vi "DB_Write.vi"(0 "Input Params":T1={"Address IP"="192.168.1.12", "Rack"=0, "Slot "=2, "DB Number"=1, "Start"=0, "Amount"=0, "Word Length"=2} {"Word Length" items=["Bit"=1, "Byte"=2, "Word"=4, "DWord"=6, "Real"=8, "Counter"=28, "Timer"=29]}, 7 "Array":u8[](array[numeric])) -> (15 "Status":string="No Error")   [LabVIEW 2023]
uses:
  snap7-full-1.4.0/LabVIEW/lib/Snap7.lvlib
panel:
  out "?":string
  out "Running":bool
  in  "?":bool
  # "DB Fill"
  # "WARNING !!!\nThis program will fill a DB Entirely"
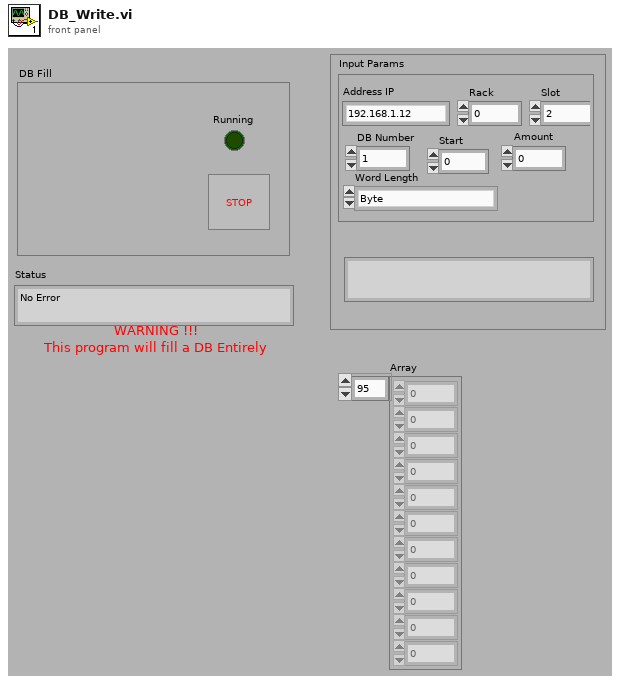
[diagram p1: front panel]
types:
  T1 = cluster{"Address IP":string, "Rack":i32, "Slot ":i32, "DB Number":i32, "Start":i32, "Amount":i32, "Word Length":i32}
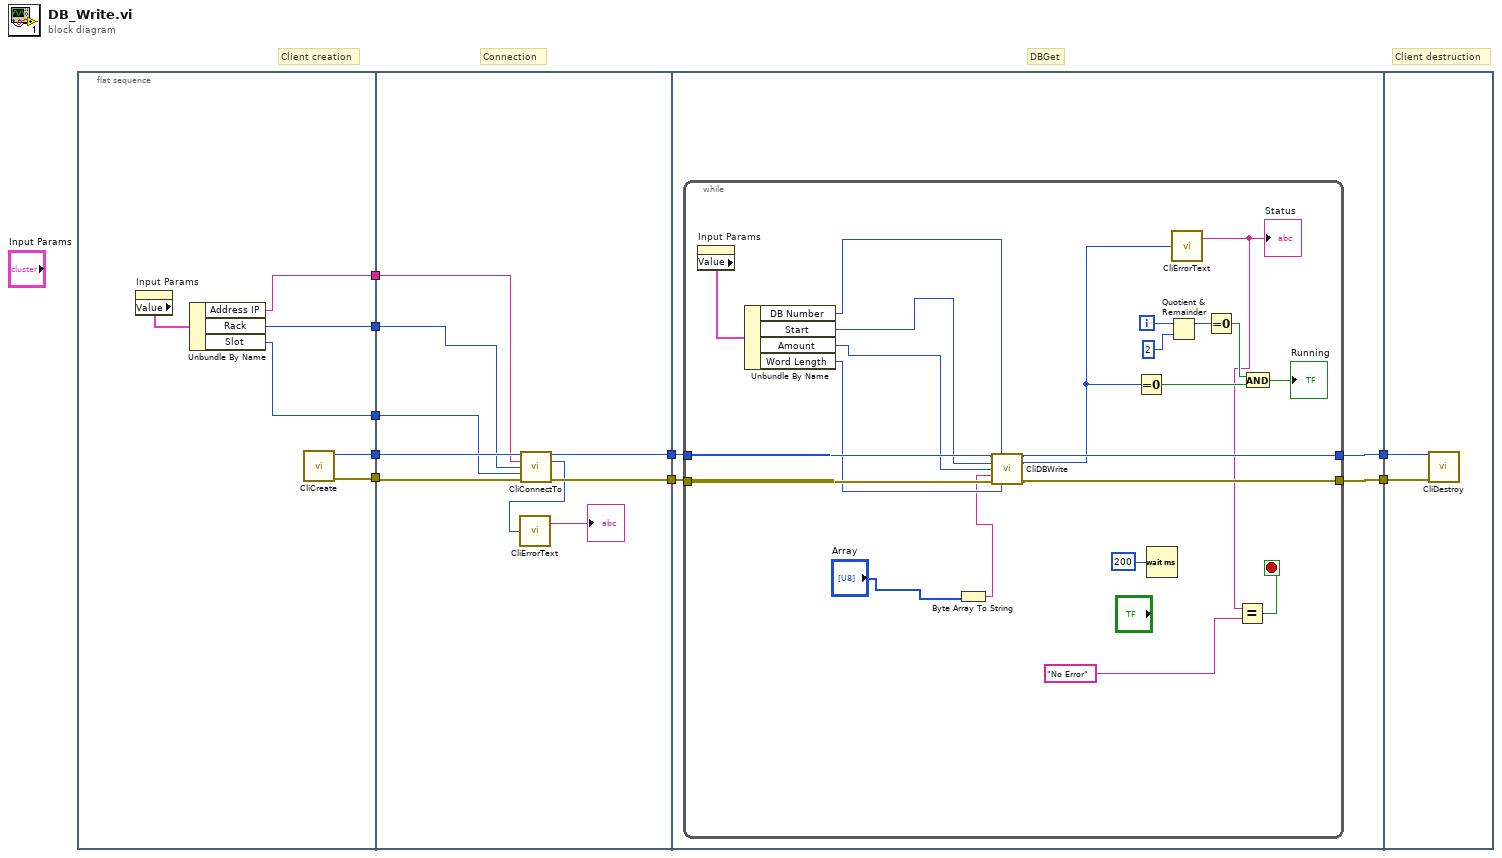
[diagram p0: block diagram]
diagram:
  # "Client destruction"
  # "DBGet"
  # "Connection"
  # "Client creation"
  n1 = flat-sequence {
    tunnel: [w15] -> w7
    tunnel: [w14] -> w6
    tunnel: [w12] -> w3
    tunnel: [w11] -> w2
    tunnel: [w10] -> w1
    tunnel: [w24] -> w9
    tunnel: [w21] -> w8
    tunnel: w7 -> [w23]
    tunnel: w6 -> [w22]
    tunnel: w3 -> [w18]
    tunnel: w2 -> [w17]
    tunnel: w1 -> [w16]
    tunnel: w9 -> [w28]
    tunnel: w8 -> [w27]
    tunnel: [w26] -> w5
    tunnel: [w25] -> w4
    tunnel: w5 -> [w52]
    tunnel: w4 -> [w51]
    frame #0 {
      n2 = property on="Input Params" class="Clust (strict)"() -> ("Value"=w13:T1)  [unwired: 2 in, 2 out]
      n3 = Unbundle By Name(w13) -> ("Address IP"=w12:string, "Rack"=w11:i32, "Slot"=w10:i32)
      n4 = call "CliCreate.vi"() -> ("ref out"=w15:u64, "error out"=w14:errorcluster)  [unwired: 14 in]
    }
    frame #1 {
      n5 = call "CliConnectTo.vi"("ref in"=w23, "Address"=w18, "Rack"=w17, "Slot"=w16, "error in (no error)"=w22) -> ("ref out"=w21:u64, "Result"=w19:i32, "error out"=w24:errorcluster)  [unwired: 8 in]
      n6 = call "CliErrorText.vi"("ErrNo"=w19) -> ("ErrMessage"=→"?":string)  [unwired: 1 out]
    }
    frame #2 {
      n7 = while {
        tunnel: w28 -> [w45]
        tunnel: w27 -> [w47]
        tunnel: [w44] -> w25
        tunnel: [w46] -> w26
        i -> [w36]
        stop <- w32 stop-if-true
        n8 = property on="Input Params" class="Clust (strict)"() -> ("Value"=w41:T1)  [unwired: 2 in, 2 out]
        n9 = Unbundle By Name(w41) -> ("DB Number"=w40:i32, "Start"=w39:i32, "Amount"=w35:i32, "Word Length"=w38:i32)
        n10 = Byte Array To String(unsigned byte array="Array") -> (string=w29:string)
        n11 = call "CliDBWrite.vi"("ref in"=w47, "DB Number"=w40, "Start"=w39, "Amount"=w35, "data in"=w29, "error in (no error)"=w45, "Word Length"=w38) -> ("ref out"=w46:u64, "Result"=w43:i32, "error out"=w44:errorcluster)  [unwired: 6 in]
        n12 = Equal To 0?(x=w43) -> (x = 0?=w34:bool)
        n13 = Wait (ms)(milliseconds to wait=u32 200 ("Loop Delay (ms)")) -> ()  [unwired: 1 out]
        n14 = Quotient & Remainder(x=w36, y=2) -> (x-y*floor(x/y)=w48:i32)  [unwired: 1 out]
        n15 = call "CliErrorText.vi"("ErrNo"=w43) -> ("ErrMessage"=w30:string)  [unwired: 1 out]
        "Status" <- w30
        n16 = Equal To 0?(x=w48) -> (x = 0?=w37:bool)
        n17 = Equal?(x=w30, y="No Error") -> (x = y?=w32:bool)
        n18 = And(x=w37, y=w34) -> (x .and. y?=→"Running":bool)
      }
    }
    frame #3 {
      n19 = call "CliDestroy.vi"("ref in"=w52, "error in (no error)"=w51) -> ()  [unwired: 13 in, 1 out]
    }
  }
